vi "Read.vi"(8 "error in (no error)":errorcluster, 11 "Agilent 344xxA in":refnum<class "Agilent 344xxA.lvclass">) -> (0 "error out":errorcluster, 1 "Unit":string, 2 "Measure":dbl, 3 "Agilent 344xxA out":refnum<class "Agilent 344xxA.lvclass">, 4 "Channel":i32)   [LabVIEW 2020, in "Agilent 344xxA.lvclass"]
uses:
  Agilent 344xxA.lvclass
  C:/Sandbox/RF Bench/Source Code/WiSpry Test Framework/Instruments/Digital Multimeter/Digital Multimeter.lvclass
  C:/Sandbox/RF Bench/Source Code/WiSpry Test Framework/Instruments/Instrument.lvclass
  Instrument.lvclass/Instrument.ctl
  <instrlib>/Agilent 34401/Public/Data/Read (Single Point).vi
  <instrlib>/Agilent 34401/Agilent 34401.lvlib
  Instrument.lvclass
  Digital Multimeter.lvclass
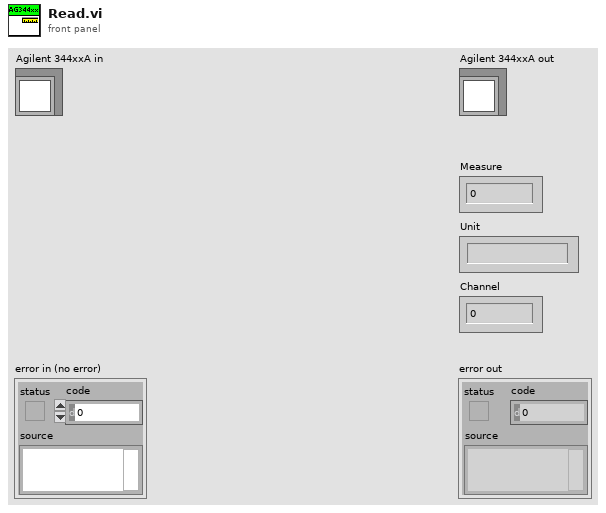
[diagram p1: front panel]
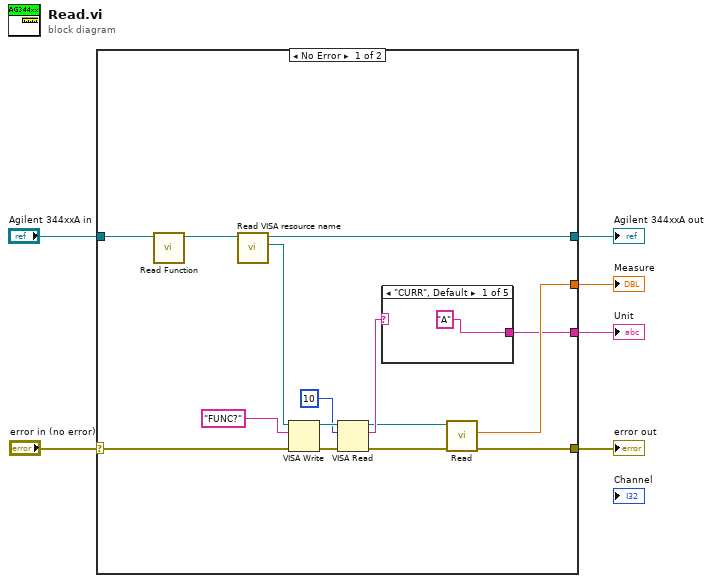
[diagram p0: block diagram]
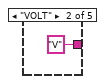
[diagram p2: hidden frame]
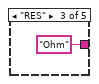
[diagram p3: hidden frame]
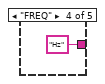
[diagram p4: hidden frame]
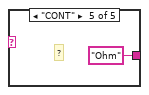
[diagram p5: hidden frame]
diagram:
  n1 = case shown="No Error" "error in (no error)" {
    selector: "error in (no error)" -> [w11 w28]
    tunnel: [w19 w28] -> w5
    tunnel: [w21 w27] -> w4
    tunnel: "Agilent 344xxA in" -> [w18 w27]
    tunnel: [w20 _] -> w2
    tunnel: [w16 _] -> w1
    frame No Error {
      n2 = call "Read Function.vi"("Digtal Multimeter in"=w18) -> ("Digtal Multimeter out"=w17:refnum<class "Agilent 344xxA.lvclass">)  [unwired: 9 in, 1 out]
      n3 = call "Read VISA resource name.vi"("Instrument in"=w17) -> ("VISA resource name"=w8:refnum<visa-resource-name>, "Instrument out"=w21:refnum<class "Agilent 344xxA.lvclass">)  [unwired: 9 in]
      n4 = VISA Write(VISA resource name=w8, write buffer="FUNC?", error in (no error)=w11) -> (VISA resource name out=w15:refnum<visa-resource-name>, error out=w14:errorcluster)  [unwired: 1 out]
      n5 = VISA Read(VISA resource name=w15, byte count=u32 10, error in (no error)=w14) -> (VISA resource name out=w7:refnum<visa-resource-name>, read buffer=w9:string, error out=w10:errorcluster)  [unwired: 1 out]
      n6 = case shown="\"CURR\", Default" w9 {
        tunnel: ["A" "V" "Ohm" "Hz" "Ohm"] -> w16
        frame "CURR", Default {
        }
        frame "VOLT" {
        }
        frame "RES" {
        }
        frame "FREQ" {
        }
        frame "CONT" {
          # "?"
        }
      }
      n7 = call-poly <instrlib>:"Read.vi"("error in (no error)"=w10, "VISA resource name"=w7) -> ("error out"=w19:errorcluster, "Measurement"=w20:dbl)  [unwired: 7 in, 1 out]
    }
    frame Error {
    }
  }
  "error out" <- w5
  "Agilent 344xxA out" <- w4
  "Measure" <- w2
  "Unit" <- w1
